vi "notify_boolean_notifier.vi"(2 "TF notifier":T1) -> (7 "notified?":bool)   [LabVIEW 2015]
uses:
  boolean_notifier.ctl
  _timing_tools_polys.lvlib
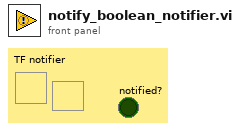
[diagram p1: front panel]
types:
  T1 = typedef "_timing_tools_polys.lvlib/boolean_notifier.ctl" = refnum<notifier>
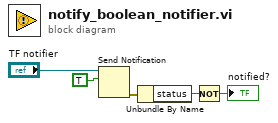
[diagram p0: block diagram]
diagram:
  n1 = Send Notification(notification=TRUE, notifier="TF notifier") -> (error out=w3:errorcluster)  [unwired: 1 in, 1 out]
  n2 = Unbundle By Name(w3) -> ("status"=w2:bool)
  n3 = Not(x=w2) -> (.not. x?=→"notified?":bool)
